vi "Set Condition for Waveform Stream (N of M Seconds).vi"(8 "error in (no error)":errorcluster, 9 "m seconds":dbl, 10 "n seconds":dbl, 11 "WaveformStreamSpecification in":T1) -> (0 "error out":errorcluster, 3 "WaveformStreamSpecification out":T1)   [LabVIEW 2020, in "NI_VS Waveform Streaming Interface.lvlib"]
doc: "Defines the condition under which NI VeriStand streams waveform data to a host computer."
uses:
  <vilib>/NI VeriStand/Execution/WaveformStreaming/NI_VS Waveform Streaming Interface.lvlib
  <vilib>/NI VeriStand/Execution/WaveformStreaming/WaveformStreamSpecification.ctl
  NationalInstruments.VeriStand.ClientAPI
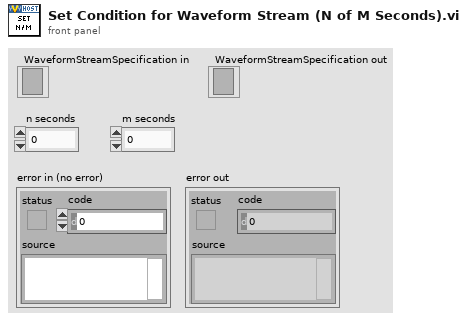
[diagram p1: front panel]
types:
  T1 = typedef "NI_VS Waveform Streaming Interface.lvlib/WaveformStreamSpecification.ctl" = refnum<k24>
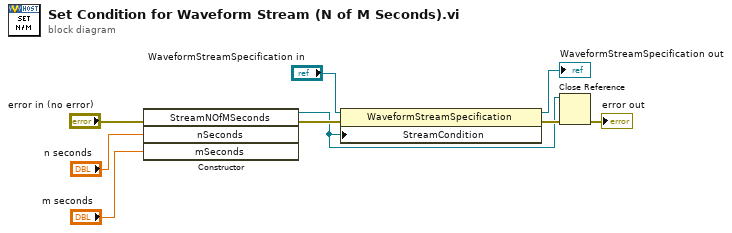
[diagram p0: block diagram]
diagram:
  n1 = constructor class="StreamNOfMSeconds"(error in="error in (no error)", "nSeconds"="n seconds", "mSeconds"="m seconds") -> (reference out=w3:refnum<k24>, error out=w5:errorcluster)  [unwired: 2 in, 3 out]
  n2 = property class="WaveformStreamSpecification"(reference="WaveformStreamSpecification in", error in=w5, "StreamCondition"=w3) -> (reference out=→"WaveformStreamSpecification out":T1, error out=w4:errorcluster)
  n3 = Close Reference(reference=w3, error in (no error)=w4) -> (error out=→"error out":errorcluster)
